vi "FTDI SPI GPIO Ini.vi"(8 "error in (no error)":errorcluster, 9 "Channel Nmb":u8, 11 "config":T1={"ClockRate"=50000, "LatencyTimer"=255, "configOptions 24-31"=0, "configOptions 16-23"=0, "configOptions 8-15"=0, "configOptions 0-7"=32, "Pin"=0, "reserved"=0} {"configOptions 24-31" format="%x"; "configOptions 16-23" format="%x"; "configOptions 8-15" format="%x"; "configOptions 0-7" format="%x"}) -> (0 "error out":errorcluster, 2 "Ini Status":bool, 3 "handle out":u32, 5 "Serial number":string, 7 "Description":string)   [LabVIEW 2018]
panel:
  # "configOptions\nThis member provides a way to enable/disable features\n\tspecific to the protocol that are implemented in the chip\n\tBIT1-0=CPOL-CPHA:\t00 - MODE0 - data captured on rising edge, propagated on falling\n \t\t\t\t\t\t01 - MODE1 - data captured on falling edge, propagated on rising\n \t\t\t\t\t\t10 - MODE2 - data captured on falling edge, propagated on rising\n \t\t\t\t\t\t11 - MODE3 - data captured on rising edge, propagated on falling\n\tBIT4-BIT2: 000 - A/B/C/D_DBUS3=ChipSelect\n\t\t\t : 001 - A/B/C/D_DBUS4=ChipSelect\n \t\t\t : 010 - A/B/C/D_DBUS5=ChipSelect\n \t\t\t : 011 - A/B/C/D_DBUS6=ChipSelect\n \t\t\t : 100 - A/B/C/D_DBUS7=ChipSelect\n \tBIT5: ChipSelect is active high if this bit is 0\n\tBIT6 -BIT31\t\t: Reserved"
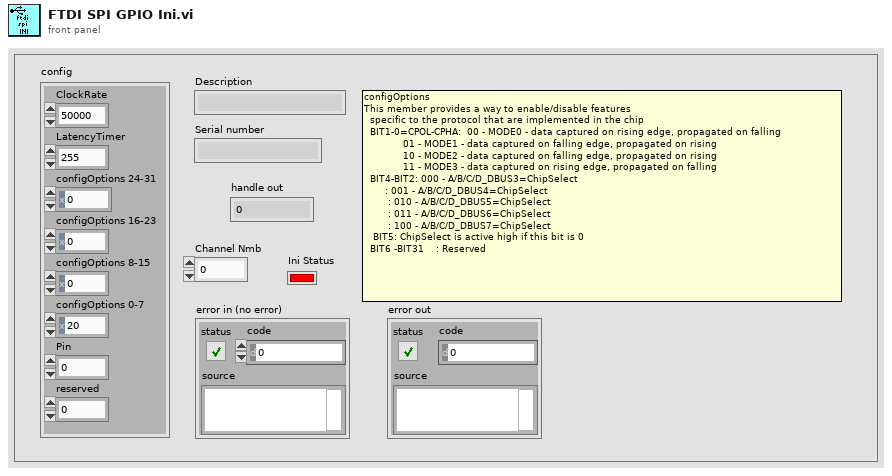
[diagram p1: front panel]
types:
  T1 = cluster{"ClockRate":u32, "LatencyTimer":u8, "configOptions 24-31":i8, "configOptions 16-23":i8, "configOptions 8-15":i8, "configOptions 0-7":u32, "Pin":u32, "reserved":u16}
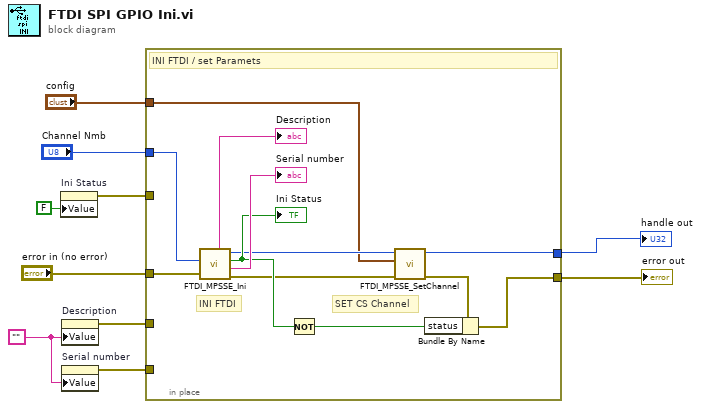
[diagram p0: block diagram]
diagram:
  w1 = ""
  n1 = property on="Ini Status" class="Bool (strict)"("Value"=FALSE ("Ini Status")) -> (error out=w5:errorcluster)  [unwired: 2 in, 1 out]
  n2 = property on="Description" class="Str"("Value"=w1) -> (error out=w3:errorcluster)  [unwired: 2 in, 1 out]
  n3 = property on="Serial number" class="Str"("Value"=w1) -> (error out=w2:errorcluster)  [unwired: 2 in, 1 out]
  n4 = in-place {
    in-place-border: [w11] -> w9
    in-place-border: [w18] -> w10
    in-place-border: "Channel Nmb" -> [w20]
    in-place-border: "config" -> [w14]
    in-place-border: "error in (no error)" -> [w19]
    in-place-border: w5 -> [_]
    in-place-border: w3 -> [_]
    in-place-border: w2 -> [_]
    # "SET CS Channel"
    # "INI FTDI"
    # "INI FTDI / set Paramets"
    n5 = call "FTDI_MPSSE_Ini.vi"("error in (no error)"=w19, "Channel Nmb"=w20) -> ("error out"=w13:errorcluster, "Serial number"=→"Serial number":string, "Ini Status"=w17:bool, "Handler"=w15:u32, "Description"=→"Description":string)  [unwired: 5 in]
    "Ini Status" <- w17
    n6 = Not(x=w17) -> (.not. x?=w16:bool)
    n7 = call "FTDI_MPSSE_SetChannel.vi"("error in (no error)"=w13, "config"=w14, "handle"=w15) -> ("error out"=w12:errorcluster, "handle out"=w11:u32)  [unwired: 7 in]
    n8 = Bundle By Name(cluster=w12, "status"=w16) -> (w18:errorcluster)
  }
  "error out" <- w10
  "handle out" <- w9
